vi "DR1 Grab and Attributes Setup.vi"() -> ()   [LabVIEW 2012]
doc: "The Grab and Attributes Setup example VI allows the user to view the current attributes and settings, update attribute settings, acquire images continuously, and display the images in an image control."
uses:
  <vilib>/userDefined/High Color/IMAQdx.ctl
  <vilib>/vision/driver/IMAQdx.llb/IMAQdx Acquisition Mode.ctl
  <vilib>/vision/driver/IMAQdx.llb/IMAQdx Buffer Number Mode.ctl
  <vilib>/vision/driver/NI_Vision_Acquisition_Software.lvlib
  Photonfocus/PFRemote/bin/pfDoubleRate.dll
panel:
  out "DoubleRate_Enable":bool
  out "Height":dbl=200.0
  out "Window_W":dbl=544.0
  out "WidthInterface":i64
  in  "Grab":bool
  out "Tooltip":string
  out "Units":string
  out "Tab Control Ref":T1
  in  "Tab Control":T2(tab)
  in  "U32 Value Control":u32(slide) scale=4.0..4044.0
  in  "DBL Value Control":dbl(slide) min=2.985074626865672 max=68.14839172363281 step=1.0 scale=2.985074626865672..68.14839172363281
  in  "String Value Control":string
  in  "Enum Value Control":u32(ring) items=["FrameStart"]
  in  "Boolean Value Control":bool=TRUE
  in  "Command Value Control":bool
  in  "Attribute Table":string(tree)
  out "Frame Rate":dbl(knob) scale=0.0..200.0 scale format="%.1f"
  out "Image":T3(plugin-control)
  out "Buffer Number":u32
  in  "Camera Name":T4
  in  "stop":bool
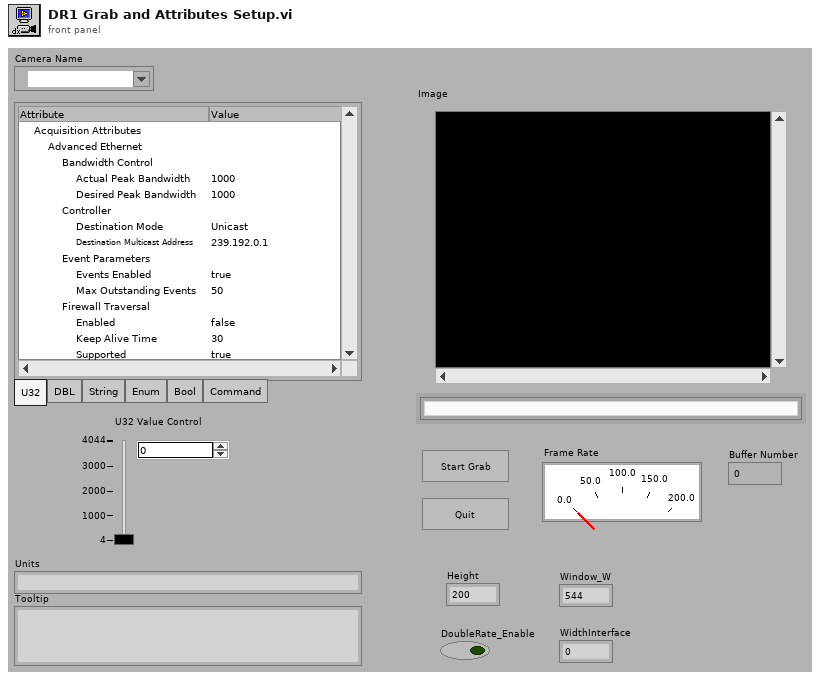
[diagram p1: front panel]
types:
  T1 = cluster{"Tab Control":refnum<vi>, "U32 Value Control":refnum<vi>, "DBL Value Control":refnum<vi>, "String Value Control":refnum<vi>, "Enum Value Control":refnum<vi>, "Boolean Value Control":refnum<vi>, "Command Value Control":refnum<vi>}
  T2 = enum32{"U32", "DBL", "String", "Enum", "Bool", "Command"}
  T3 = typedef "IMAQ Image.ctl" = refnum<image>
  T4 = typedef "IMAQdx.ctl" = refnum<k21>
  T5 = typedef "NI_Vision_Acquisition_Software.lvlib/IMAQdx Acquisition Mode.ctl" = enum32{"One Shot", "Continuous"}
  T6 = typedef "NI_Vision_Acquisition_Software.lvlib/IMAQdx Buffer Number Mode.ctl" = enum32{"Next", "Last", "Buffer Number"}
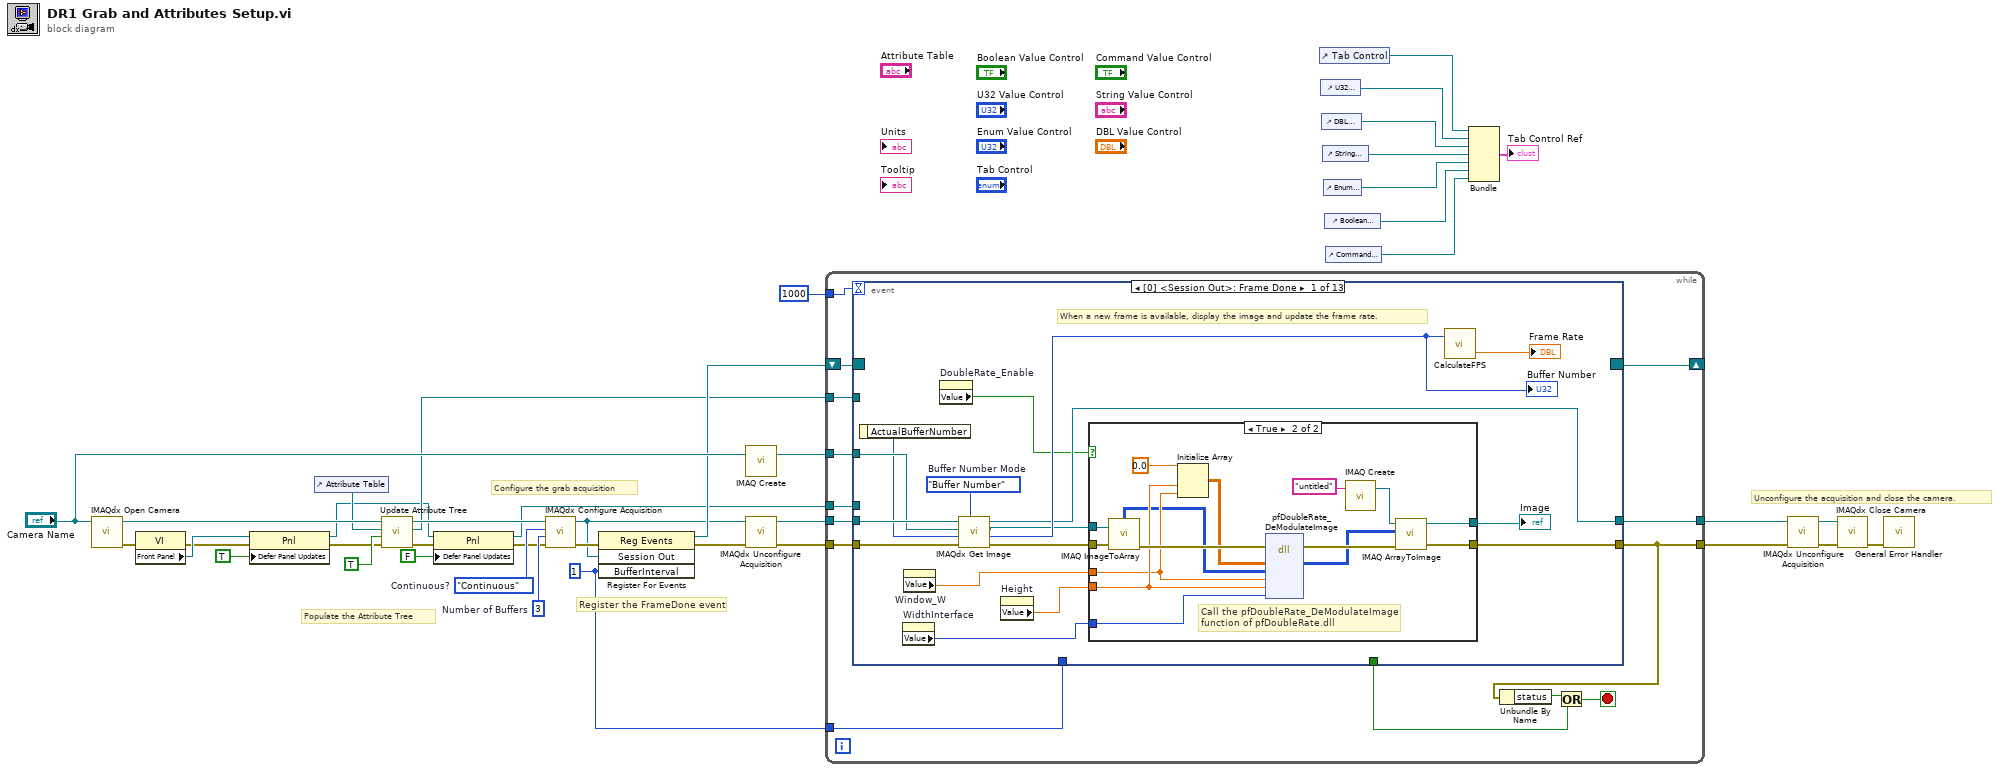
[diagram p0: block diagram]
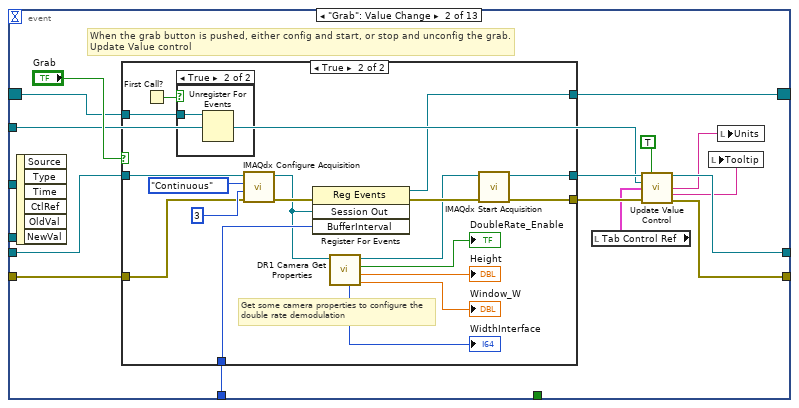
[diagram p3: hidden frame]
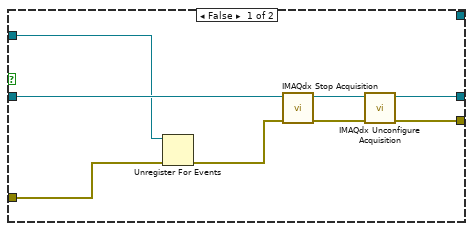
[diagram p4: hidden frame]
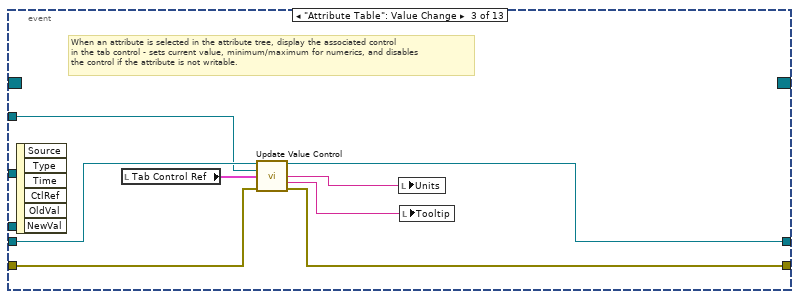
[diagram p6: hidden frame]
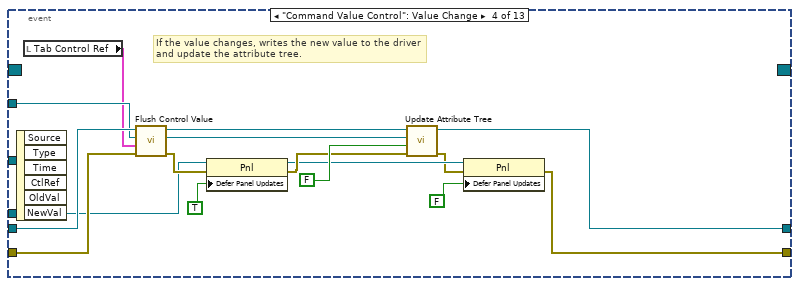
[diagram p7: hidden frame]
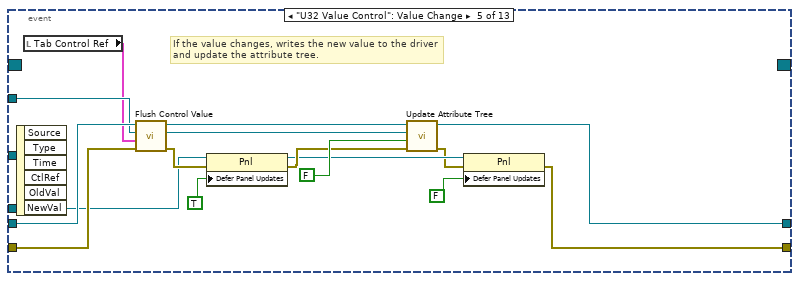
[diagram p8: hidden frame]
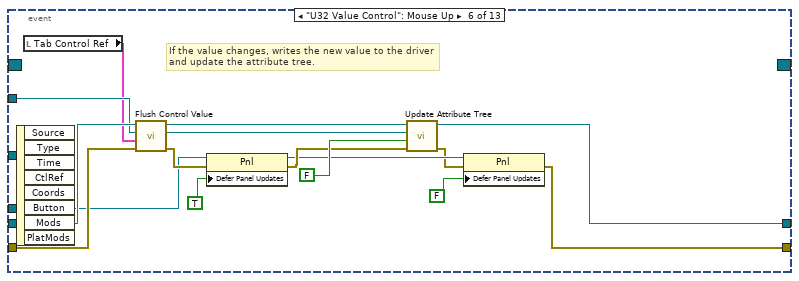
[diagram p9: hidden frame]
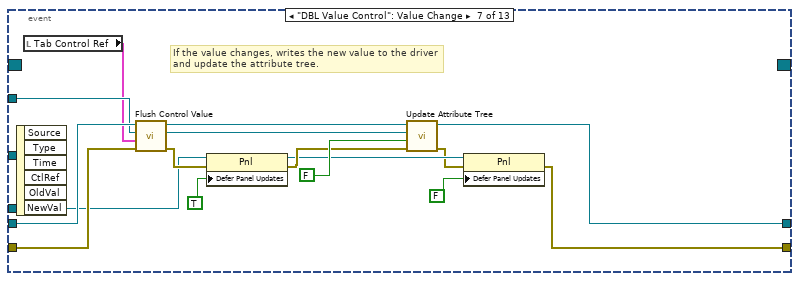
[diagram p10: hidden frame]
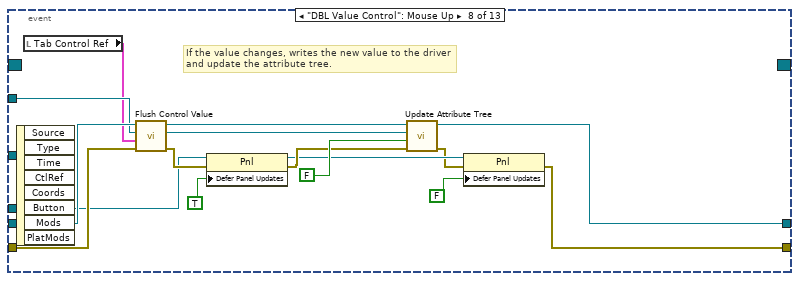
[diagram p11: hidden frame]
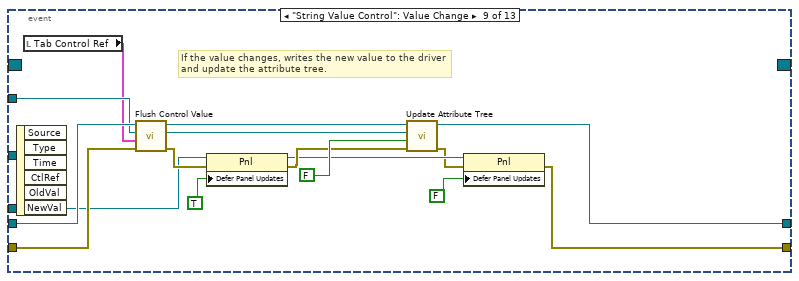
[diagram p12: hidden frame]
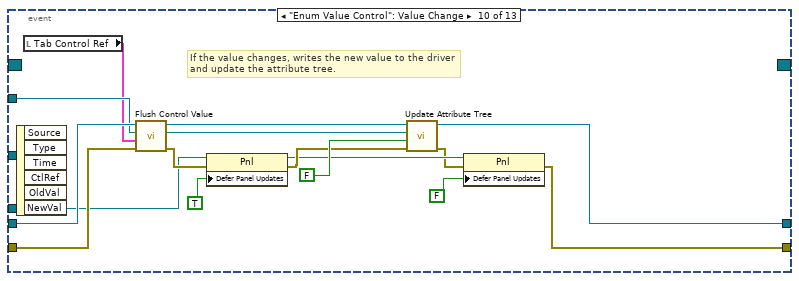
[diagram p13: hidden frame]
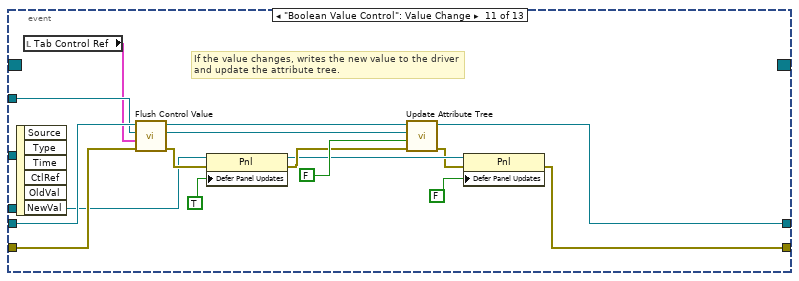
[diagram p14: hidden frame]
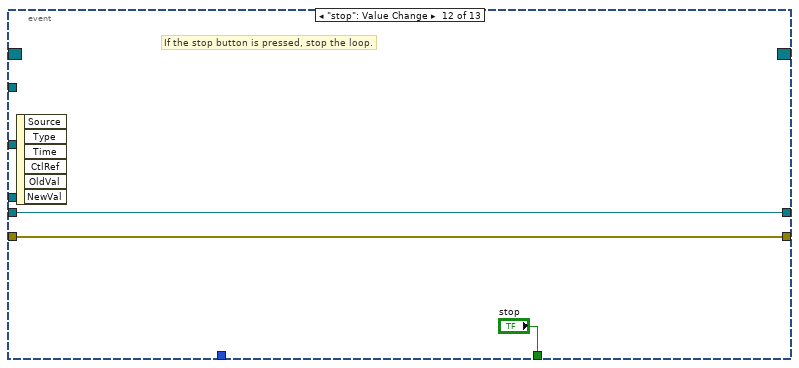
[diagram p15: hidden frame]
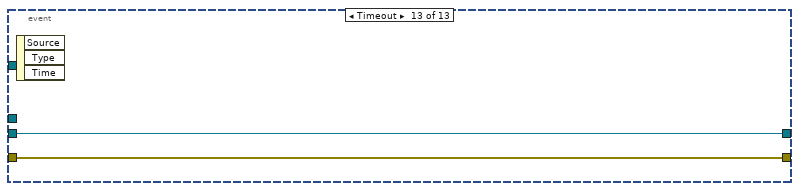
[diagram p16: hidden frame]
diagram:
  w5 = u32 1 ("BufferInterval")
  w36 = u32 3  # Number of Buffers
  w37 = IMAQdx_Acquisition_Mode."Continuous"  # Continuous?
  # "Unconfigure the acquisition and close the camera."
  # "Register the FrameDone event"
  # "Configure the grab acquisition"
  # "Populate the Attribute Tree"
  n1 = call <vilib>:"IMAQdx Open Camera.vi"("Session In"="Camera Name") -> ("error out"=w8:errorcluster, "Session Out"=w22:T4)  [unwired: 2 in, 7 out]
  n2 = property class="VI"(error in=w8) -> (error out=w9:errorcluster, "Front Panel"=w10:refnum<vi>)  [unwired: 1 in, 1 out]
  n3 = property class="Pnl"(reference=w10, error in=w9, "Defer Panel Updates"=TRUE) -> (reference out=w13:refnum<vi>, error out=w17:errorcluster)
  n4 = control-ref of="Attribute Table"() -> (w20:refnum<vi>)
  n5 = call <userlib>:"Update Attribute Tree.vi"("error in"=w17, "Flush Tree?"=TRUE, "Tree Control In"=w20, "Camera Name In"=w22) -> ("error out"=w16:errorcluster, "Tree Control Out"=w18:refnum<vi>, "Session Out"=w21:T4)  [unwired: 1 out]
  n6 = property class="Pnl"(reference=w13, error in=w16, "Defer Panel Updates"=FALSE) -> (reference out=w12:refnum<vi>, error out=w14:errorcluster)
  n7 = call <vilib>:"IMAQdx Configure Acquisition.vi"("error in"=w14, "Number of Buffers"=w36, "Continuous?"=w37, "Session In"=w21) -> ("error out"=w33:errorcluster, "Session Out"=w2:T4)  [unwired: 6 out]
  n8 = register-events(error in=w33, w2, w5) -> (reference out=w32:refnum<event-registration>, error out=w4:errorcluster)  [unwired: 1 in]
  n9 = call "IMAQ Create"("Image Name"="Camera Name") -> ("New Image"=w40:T3)  [unwired: 3 in, 2 out]
  n10 = call <vilib>:"IMAQdx Unconfigure Acquisition.vi"("error in"=w4, "Session In"=w2) -> ("error out"=w3:errorcluster, "Session Out"=w1:T4)  [unwired: 8 out]
  n11 = while {
    tunnel: [w49] -> w7
    tunnel: w3 -> [w51]
    tunnel: w1 -> [w52]
    tunnel: [w48] -> w6
    tunnel: w40 -> [w50]
    tunnel: 1000 -> [w46]
    tunnel: w18 -> [w45]
    tunnel: w12 -> [w44]
    tunnel: w5 -> [w42]
    shift-right: [w41] -> _
    shift-left: w32 -> [w47]
    stop <- w54 stop-if-true
    n12 = event shown="[0] <Session Out>: Frame Done" {
      selector: w47 -> [_ w99 _ _ _ _ _ _ _ _ _ _ _]
      dyn-events: [_ w101 _ _ _ _ _ _ _ _ _ _ _] -> w41
      timeout: w46 -> [_ _ _ _ _ _ _ _ _ _ _ _ _]
      tunnel: w52 -> [w70 w88 w137 w152 w168 w184 w200 w216 w232 w248 w264 w267 w269]
      tunnel: w51 -> [w69 w98 w135 w153 w169 w185 w201 w217 w233 w249 w265 w266 w270]
      tunnel: w50 -> [w68 _ _ _ _ _ _ _ _ _ _ _ _]
      tunnel: [w60 w96 w136 w138 w154 w170 w186 w202 w218 w234 w250 w267 w269] -> w49
      tunnel: [w61 w94 w134 w139 w155 w171 w187 w203 w219 w235 w251 w266 w270] -> w48
      tunnel: w45 -> [_ w92 w130 w150 w166 w182 w198 w214 w230 w246 w262 _ _]
      tunnel: w44 -> [_ _ _ w144 w160 w176 w192 w208 w224 w240 w256 _ _]
      tunnel: [_ _ _ _ _ _ _ _ _ _ _ "stop" _] -> w43
      tunnel: w42 -> [_ w100 _ _ _ _ _ _ _ _ _ _ _]
      event event #0x0 {
        w66 = IMAQdx_Buffer_Number_Mode."Buffer Number"  # Buffer Number Mode
        # "When a new frame is available, display the image and update the frame rate."
        n13 = event-data() -> ("ActualBufferNumber"=w65:u32)  [unwired: 1 out]
        n14 = property on="WidthInterface" class="DigNum (strict)"() -> ("Value"=w57:i64)  [unwired: 2 in, 2 out]
        n15 = property on="Window_W" class="DigNum (strict)"() -> ("Value"=w56:dbl)  [unwired: 2 in, 2 out]
        n16 = property on="DoubleRate_Enable" class="Bool (strict)"() -> ("Value"=w58:bool)  [unwired: 2 in, 2 out]
        n17 = call <vilib>:"IMAQdx Get Image.vi"("Buffer Number Mode (Next)"=w66, "error in"=w69, "Buffer Number In"=w65, "Image In"=w68, "Session In"=w70) -> ("error out"=w63:errorcluster, "Buffer Number Out"=w64:u32, "Image Out"=w59:T3, "Session Out"=w60:T4)  [unwired: 3 out]
        "Buffer Number" <- w64
        n18 = property on="Height" class="DigNum (strict)"() -> ("Value"=w55:dbl)  [unwired: 2 in, 2 out]
        n19 = case shown="True" w58 {
          tunnel: w63 -> [w72 w85]
          tunnel: [w71 w84] -> w62
          tunnel: [w72 w83] -> w61
          tunnel: w57 -> [_ w80]
          tunnel: w55 -> [_ w79]
          tunnel: w59 -> [w71 w78]
          tunnel: w56 -> [_ w74]
          frame False {
          }
          frame True {
            # "Call the pfDoubleRate_DeModulateImage \nfunction of pfDoubleRate.dll"
            n20 = call "IMAQ ImageToArray"("error in (no error)"=w85, "Image"=w78) -> ("error out"=w86:errorcluster, "Image Pixels (U8)"=w73:u8[][])  [unwired: 2 in, 3 out]
            n21 = Initialize Array "Initialize Array"(0.0 ("element"), w79, w74) -> (w81:dbl[][])
            n22 = dll-call lib="C:/Program Files/Photonfocus/PFRemote/bin/pfDoubleRate.dll" fn="pfDoubleRate_DeModulateImage"(error in=w86, "Image"=w81, "modImage"=w73, "Width"=w74, "Height"=w79, "modWidth"=w80) -> (error out=w87:errorcluster, "Image"=w75:u8[][])  [unwired: 7 in, 1 out]
            n23 = call "IMAQ Create"("Image Name"="untitled") -> ("New Image"=w77:T3)  [unwired: 4 in, 1 out]
            n24 = call "IMAQ ArrayToImage"("error in (no error)"=w87, "Image Pixels (U8)"=w75, "Image"=w77) -> ("error out"=w83:errorcluster, "Image Out"=w84:T3)  [unwired: 7 in]
          }
        }
        "Image" <- w62
        n25 = call <userlib>:"CalculateFPS.vi"("buffer number"=w64) -> ("processed FPS"=→"Frame Rate":dbl)  [unwired: 2 out]
      }
      event "Grab": Value Change {
        # "When the grab button is pushed, either config and start, or stop and unconfig the grab.\nUpdate Value control"
        n26 = event-data() -> ()  [unwired: 7 out]
        n27 = case shown="True" "Grab" {
          tunnel: w88 -> [w110 w117]
          tunnel: [w107 w128] -> w97
          tunnel: [w106 w127] -> w95
          tunnel: [_ w122] -> w101
          tunnel: w100 -> [_ w121]
          tunnel: w99 -> [w105 w119]
          tunnel: w98 -> [w103 w120]
          frame False {
            n28 = Unregister For Events(event registration refnum=w105, error in=w103) -> (error out=w104:errorcluster)
            n29 = call <vilib>:"IMAQdx Stop Acquisition.vi"("error in"=w104, "Session In"=w110) -> ("error out"=w108:errorcluster, "Session Out"=w109:T4)  [unwired: 8 out]
            n30 = call <vilib>:"IMAQdx Unconfigure Acquisition.vi"("error in"=w108, "Session In"=w109) -> ("error out"=w106:errorcluster, "Session Out"=w107:T4)  [unwired: 8 out]
          }
          frame True {
            # "Get some camera properties to configure the double rate demodulation"
            n31 = First Call?() -> (First Call?: T/F=w118:bool)
            n32 = case shown="True" w118 {
              tunnel: w119 -> [_ w129]
              frame False {
              }
              frame True {
                n33 = Unregister For Events(event registration refnum=w129) -> ()  [unwired: 1 in, 1 out]
              }
            }
            n34 = call <vilib>:"IMAQdx Configure Acquisition.vi"("error in"=w120, "Number of Buffers"=u32 3, "Continuous?"=IMAQdx_Acquisition_Mode."Continuous", "Session In"=w117) -> ("error out"=w124:errorcluster, "Session Out"=w116:T4)  [unwired: 6 out]
            n35 = register-events(error in=w124, w116, w121) -> (reference out=w122:refnum<event-registration>, error out=w123:errorcluster)  [unwired: 1 in]
            n36 = call "DR1 Camera Get Properties.vi"("Session In"=w116) -> ("Window_W"=→"Window_W":dbl, "Height"=→"Height":dbl, "DoubleRate_Enable"=→"DoubleRate_Enable":bool, "Session Out"=w115:T4, "WidthInterface"=→"WidthInterface":i64)  [unwired: 4 in]
            n37 = call <vilib>:"IMAQdx Start Acquisition.vi"("error in"=w123, "Session In"=w115) -> ("error out"=w127:errorcluster, "Session Out"=w128:T4)  [unwired: 8 out]
          }
        }
        n38 = local read "Tab Control Ref"() -> (w93:T1)
        n39 = call <userlib>:"Update Value Control.vi"("Session In"=w97, "Force update?"=TRUE, "Tree Control In"=w92, "Tab Control Ref In"=w93, "error in (no error)"=w95) -> ("Session Out"=w96:T4, "Units"=w91:string, "Tooltip"=w90:string, "error out"=w94:errorcluster)  [unwired: 7 out]
        n40 = local write "Tooltip"(w90) -> ()
        n41 = local write "Units"(w91) -> ()
      }
      event "Attribute Table": Value Change {
        # "When an attribute is selected in the attribute tree, display the associated control\nin the tab control - sets current value, minimum/maximum for numerics, and disables\nthe control if the attribute is not writable."
        n42 = event-data() -> ()  [unwired: 7 out]
        n43 = local read "Tab Control Ref"() -> (w133:T1)
        n44 = call <userlib>:"Update Value Control.vi"("Session In"=w137, "Tree Control In"=w130, "Tab Control Ref In"=w133, "error in (no error)"=w135) -> ("Session Out"=w136:T4, "Units"=w132:string, "Tooltip"=w131:string, "error out"=w134:errorcluster)  [unwired: 1 in, 7 out]
        n45 = local write "Units"(w132) -> ()
        n46 = local write "Tooltip"(w131) -> ()
      }
      event "Command Value Control": Value Change {
        # "If the value changes, writes the new value to the driver\nand update the attribute tree."
        n47 = event-data() -> ()  [unwired: 7 out]
        n48 = local read "Tab Control Ref"() -> (w149:T1)
        n49 = call <userlib>:"Flush Control Value.vi"("error in (no error)"=w153, "Tab Control Ref In"=w149, "Tree Control In"=w150, "Session In"=w152) -> ("error out"=w145:errorcluster, "Tree Control Out"=w148:refnum<vi>, "Session Out"=w151:T4)  [unwired: 1 out]
        n50 = property class="Pnl"(reference=w144, error in=w145, "Defer Panel Updates"=TRUE) -> (reference out=w142:refnum<vi>, error out=w146:errorcluster)
        n51 = call <userlib>:"Update Attribute Tree.vi"("error in"=w146, "Flush Tree?"=FALSE, "Tree Control In"=w148, "Camera Name In"=w151) -> ("error out"=w141:errorcluster, "Session Out"=w138:T4)  [unwired: 2 out]
        n52 = property class="Pnl"(reference=w142, error in=w141, "Defer Panel Updates"=FALSE) -> (error out=w139:errorcluster)  [unwired: 1 out]
      }
      event "U32 Value Control": Value Change {
        # "If the value changes, writes the new value to the driver\nand update the attribute tree."
        n53 = event-data() -> ()  [unwired: 7 out]
        n54 = local read "Tab Control Ref"() -> (w165:T1)
        n55 = call <userlib>:"Flush Control Value.vi"("error in (no error)"=w169, "Tab Control Ref In"=w165, "Tree Control In"=w166, "Session In"=w168) -> ("error out"=w161:errorcluster, "Tree Control Out"=w164:refnum<vi>, "Session Out"=w167:T4)  [unwired: 1 out]
        n56 = property class="Pnl"(reference=w160, error in=w161, "Defer Panel Updates"=TRUE) -> (reference out=w158:refnum<vi>, error out=w162:errorcluster)
        n57 = call <userlib>:"Update Attribute Tree.vi"("error in"=w162, "Flush Tree?"=FALSE, "Tree Control In"=w164, "Camera Name In"=w167) -> ("error out"=w157:errorcluster, "Session Out"=w154:T4)  [unwired: 2 out]
        n58 = property class="Pnl"(reference=w158, error in=w157, "Defer Panel Updates"=FALSE) -> (error out=w155:errorcluster)  [unwired: 1 out]
      }
      event "U32 Value Control": Mouse Up {
        # "If the value changes, writes the new value to the driver\nand update the attribute tree."
        n59 = event-data() -> ()  [unwired: 9 out]
        n60 = local read "Tab Control Ref"() -> (w181:T1)
        n61 = call <userlib>:"Flush Control Value.vi"("error in (no error)"=w185, "Tab Control Ref In"=w181, "Tree Control In"=w182, "Session In"=w184) -> ("error out"=w177:errorcluster, "Tree Control Out"=w180:refnum<vi>, "Session Out"=w183:T4)  [unwired: 1 out]
        n62 = property class="Pnl"(reference=w176, error in=w177, "Defer Panel Updates"=TRUE) -> (reference out=w174:refnum<vi>, error out=w178:errorcluster)
        n63 = call <userlib>:"Update Attribute Tree.vi"("error in"=w178, "Flush Tree?"=FALSE, "Tree Control In"=w180, "Camera Name In"=w183) -> ("error out"=w173:errorcluster, "Session Out"=w170:T4)  [unwired: 2 out]
        n64 = property class="Pnl"(reference=w174, error in=w173, "Defer Panel Updates"=FALSE) -> (error out=w171:errorcluster)  [unwired: 1 out]
      }
      event "DBL Value Control": Value Change {
        # "If the value changes, writes the new value to the driver\nand update the attribute tree."
        n65 = event-data() -> ()  [unwired: 7 out]
        n66 = local read "Tab Control Ref"() -> (w197:T1)
        n67 = call <userlib>:"Flush Control Value.vi"("error in (no error)"=w201, "Tab Control Ref In"=w197, "Tree Control In"=w198, "Session In"=w200) -> ("error out"=w193:errorcluster, "Tree Control Out"=w196:refnum<vi>, "Session Out"=w199:T4)  [unwired: 1 out]
        n68 = property class="Pnl"(reference=w192, error in=w193, "Defer Panel Updates"=TRUE) -> (reference out=w190:refnum<vi>, error out=w194:errorcluster)
        n69 = call <userlib>:"Update Attribute Tree.vi"("error in"=w194, "Flush Tree?"=FALSE, "Tree Control In"=w196, "Camera Name In"=w199) -> ("error out"=w189:errorcluster, "Session Out"=w186:T4)  [unwired: 2 out]
        n70 = property class="Pnl"(reference=w190, error in=w189, "Defer Panel Updates"=FALSE) -> (error out=w187:errorcluster)  [unwired: 1 out]
      }
      event "DBL Value Control": Mouse Up {
        # "If the value changes, writes the new value to the driver\nand update the attribute tree."
        n71 = event-data() -> ()  [unwired: 9 out]
        n72 = local read "Tab Control Ref"() -> (w213:T1)
        n73 = call <userlib>:"Flush Control Value.vi"("error in (no error)"=w217, "Tab Control Ref In"=w213, "Tree Control In"=w214, "Session In"=w216) -> ("error out"=w209:errorcluster, "Tree Control Out"=w212:refnum<vi>, "Session Out"=w215:T4)  [unwired: 1 out]
        n74 = property class="Pnl"(reference=w208, error in=w209, "Defer Panel Updates"=TRUE) -> (reference out=w206:refnum<vi>, error out=w210:errorcluster)
        n75 = call <userlib>:"Update Attribute Tree.vi"("error in"=w210, "Flush Tree?"=FALSE, "Tree Control In"=w212, "Camera Name In"=w215) -> ("error out"=w205:errorcluster, "Session Out"=w202:T4)  [unwired: 2 out]
        n76 = property class="Pnl"(reference=w206, error in=w205, "Defer Panel Updates"=FALSE) -> (error out=w203:errorcluster)  [unwired: 1 out]
      }
      event "String Value Control": Value Change {
        # "If the value changes, writes the new value to the driver\nand update the attribute tree."
        n77 = event-data() -> ()  [unwired: 7 out]
        n78 = local read "Tab Control Ref"() -> (w229:T1)
        n79 = call <userlib>:"Flush Control Value.vi"("error in (no error)"=w233, "Tab Control Ref In"=w229, "Tree Control In"=w230, "Session In"=w232) -> ("error out"=w225:errorcluster, "Tree Control Out"=w228:refnum<vi>, "Session Out"=w231:T4)  [unwired: 1 out]
        n80 = property class="Pnl"(reference=w224, error in=w225, "Defer Panel Updates"=TRUE) -> (reference out=w222:refnum<vi>, error out=w226:errorcluster)
        n81 = call <userlib>:"Update Attribute Tree.vi"("error in"=w226, "Flush Tree?"=FALSE, "Tree Control In"=w228, "Camera Name In"=w231) -> ("error out"=w221:errorcluster, "Session Out"=w218:T4)  [unwired: 2 out]
        n82 = property class="Pnl"(reference=w222, error in=w221, "Defer Panel Updates"=FALSE) -> (error out=w219:errorcluster)  [unwired: 1 out]
      }
      event "Enum Value Control": Value Change {
        # "If the value changes, writes the new value to the driver\nand update the attribute tree."
        n83 = event-data() -> ()  [unwired: 7 out]
        n84 = local read "Tab Control Ref"() -> (w245:T1)
        n85 = call <userlib>:"Flush Control Value.vi"("error in (no error)"=w249, "Tab Control Ref In"=w245, "Tree Control In"=w246, "Session In"=w248) -> ("error out"=w241:errorcluster, "Tree Control Out"=w244:refnum<vi>, "Session Out"=w247:T4)  [unwired: 1 out]
        n86 = property class="Pnl"(reference=w240, error in=w241, "Defer Panel Updates"=TRUE) -> (reference out=w238:refnum<vi>, error out=w242:errorcluster)
        n87 = call <userlib>:"Update Attribute Tree.vi"("error in"=w242, "Flush Tree?"=FALSE, "Tree Control In"=w244, "Camera Name In"=w247) -> ("error out"=w237:errorcluster, "Session Out"=w234:T4)  [unwired: 2 out]
        n88 = property class="Pnl"(reference=w238, error in=w237, "Defer Panel Updates"=FALSE) -> (error out=w235:errorcluster)  [unwired: 1 out]
      }
      event "Boolean Value Control": Value Change {
        # "If the value changes, writes the new value to the driver\nand update the attribute tree."
        n89 = event-data() -> ()  [unwired: 7 out]
        n90 = local read "Tab Control Ref"() -> (w261:T1)
        n91 = call <userlib>:"Flush Control Value.vi"("error in (no error)"=w265, "Tab Control Ref In"=w261, "Tree Control In"=w262, "Session In"=w264) -> ("error out"=w257:errorcluster, "Tree Control Out"=w260:refnum<vi>, "Session Out"=w263:T4)  [unwired: 1 out]
        n92 = property class="Pnl"(reference=w256, error in=w257, "Defer Panel Updates"=TRUE) -> (reference out=w254:refnum<vi>, error out=w258:errorcluster)
        n93 = call <userlib>:"Update Attribute Tree.vi"("error in"=w258, "Flush Tree?"=FALSE, "Tree Control In"=w260, "Camera Name In"=w263) -> ("error out"=w253:errorcluster, "Session Out"=w250:T4)  [unwired: 2 out]
        n94 = property class="Pnl"(reference=w254, error in=w253, "Defer Panel Updates"=FALSE) -> (error out=w251:errorcluster)  [unwired: 1 out]
      }
      event "stop": Value Change {
        # "If the stop button is pressed, stop the loop."
        n95 = event-data() -> ()  [unwired: 7 out]
      }
      event Timeout {
        n96 = event-data() -> ()  [unwired: 4 out]
      }
    }
    n97 = Unbundle By Name(w48) -> ("status"=w53:bool)
    n98 = Or(x=w53, y=w43) -> (x .or. y?=w54:bool)
  }
  n99 = control-ref of="Tab Control"() -> (w30:refnum<vi>)
  n100 = control-ref of="U32 Value Control"() -> (w28:refnum<vi>)
  n101 = control-ref of="DBL Value Control"() -> (w27:refnum<vi>)
  n102 = control-ref of="String Value Control"() -> (w29:refnum<vi>)
  n103 = control-ref of="Enum Value Control"() -> (w26:refnum<vi>)
  n104 = control-ref of="Boolean Value Control"() -> (w25:refnum<vi>)
  n105 = control-ref of="Command Value Control"() -> (w24:refnum<vi>)
  n106 = Bundle("Tab Control"=w30, "U32 Value Control"=w28, "DBL Value Control"=w27, "String Value Control"=w29, "Enum Value Control"=w26, "Boolean Value Control"=w25, "Command Value Control"=w24) -> (→"Tab Control Ref":T1)  [unwired: 1 out]
  n107 = call <vilib>:"IMAQdx Unconfigure Acquisition.vi"("error in"=w6, "Session In"=w7) -> ("error out"=w35:errorcluster, "Session Out"=w34:T4)  [unwired: 8 out]
  n108 = call <vilib>:"IMAQdx Close Camera.vi"("error in"=w35, "Session In"=w34) -> ("error out"=w39:errorcluster)  [unwired: 9 out]
  n109 = call <vilib>:"General Error Handler.vi"("error in (no error)"=w39) -> ()  [unwired: 1 in, 14 out]
